vi "scale.vi"() -> ()   [LabVIEW 2016]
panel:
  out "Scale":dbl(knob) scale=0.0..150.0
  out "kg":dbl
  out "data":dbl
  out "Waveform Chart":dbl[](graph)
  in  "stop":bool
  out "median":dbl
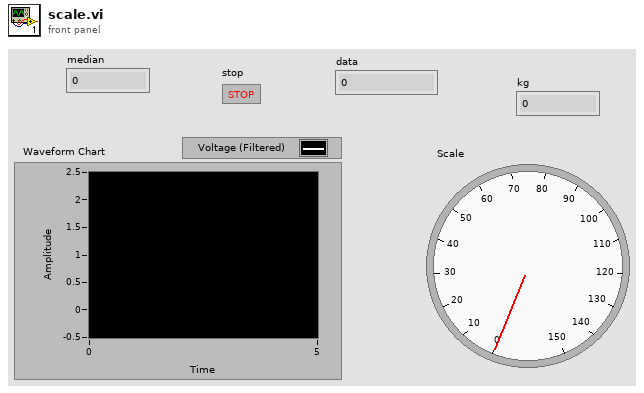
[diagram p1: front panel]
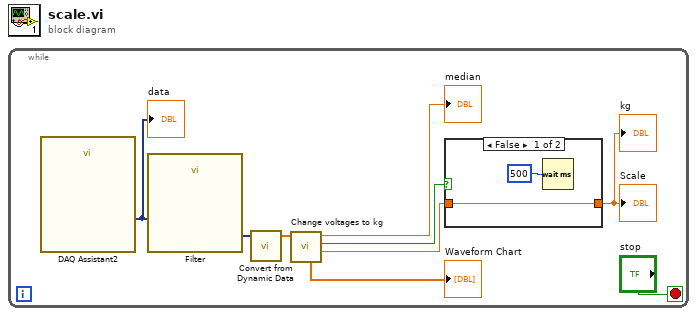
[diagram p0: block diagram]
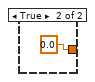
[diagram p2: hidden frame]
diagram:
  n1 = while {
    stop <- "stop" stop-if-true
    n2 = call "DAQ Assistant2"() -> ("data"=w8:dynamicdata)  [unwired: 17 in, 2 out]
    "data" <- w8
    n3 = call "Filter"("Signal"=w8) -> ("Filtered Signal"=w7:dynamicdata)  [unwired: 9 in, 1 out]
    n4 = call "Convert from Dynamic Data"("Dynamic Data Type"=w7) -> ("Array"=w9:dbl[])  [unwired: 3 in]
    n5 = call "Change voltages to kg.vi"("Array"=w9) -> ("Numeric"=w4:dbl, "Boolean"=w6:bool, "Numeric 2"=→"median":dbl, "Waveform Chart"=→"Waveform Chart":dbl[])  [unwired: 7 in]
    n6 = case shown="False" w6 {
      tunnel: w4 -> [w11 _]
      tunnel: [w11 0.0] -> w2
      frame False {
        n7 = Wait (ms)(milliseconds to wait=u32 500) -> ()  [unwired: 1 out]
      }
      frame True {
      }
    }
    "kg" <- w2
    "Scale" <- w2
  }
